vi "获得信号的最大幅值及对应的相位和频率.vi"(0 "信号":waveform(dbl)) -> (1 "max（f)":dbl, 2 "max幅值":dbl, 3 "max相位":dbl, 4 "幅值+ i相位":cdb)   [LabVIEW 2014]
uses:
  <vilib>/express/express analysis/Spectral/Block/exnSpectralBlock spectral measurements peak poly.vi
  <vilib>/express/express analysis/Spectral/Block/exnSpectralBlock spectral measurements peak WFM.vi
  <vilib>/express/express analysis/Spectral/XNode/ExpressSpectralMeasurementsBlockNode.xnode
panel:
  out "r":dbl
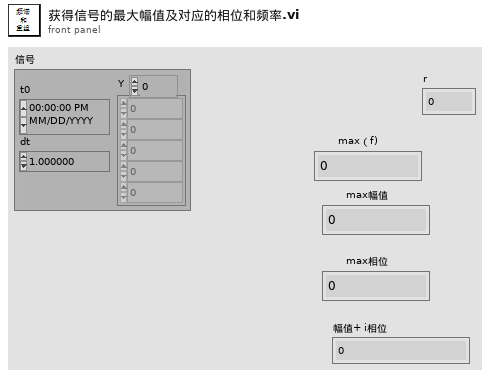
[diagram p1: front panel]
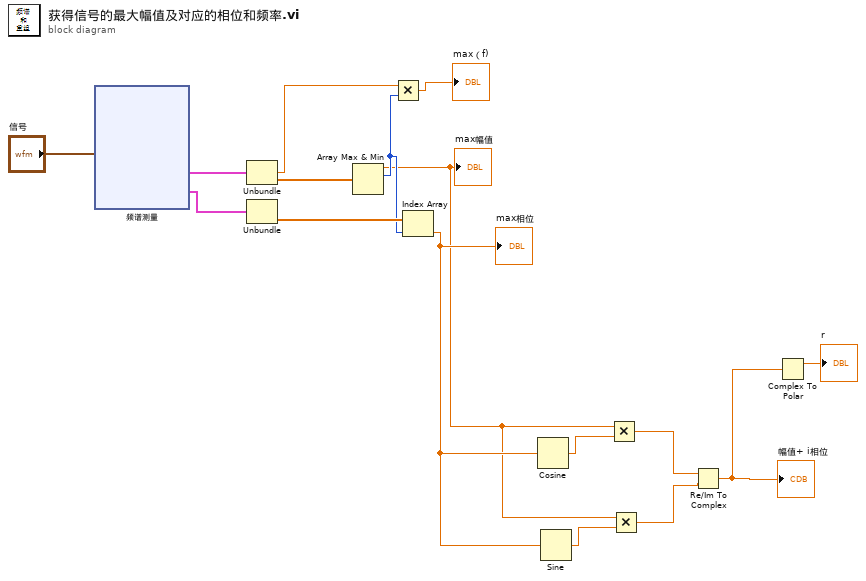
[diagram p0: block diagram]
diagram:
  n1 = xnode "频谱测量"("信号"="信号") -> ("FFT - （峰值）"=w16:cluster{"f0":dbl, "df":dbl, "magnitude":dbl[]}, "相位"=w15:cluster{"f0":dbl, "df":dbl, "phase":dbl[]})  [unwired: 1 in, 1 out]
  n2 = Unbundle(w16) -> ("df"=w13:dbl, "magnitude"=w14:dbl[])  [unwired: 1 out]
  n3 = Unbundle(w15) -> ("phase"=w11:dbl[])  [unwired: 2 out]
  n4 = Array Max & Min(array=w14) -> (max value=w6:dbl, max index (indices)=w10:i32)  [unwired: 2 out]
  "max幅值" <- w6
  n5 = Multiply(x=w13, y=w10) -> (x*y=→"max（f)":dbl)
  n6 = Index Array(array=w11, index=w10) -> (element=w9:dbl)
  "max相位" <- w9
  n7 = Cosine(x=w9) -> (cos(x)=w8:dbl)
  n8 = Sine(x=w9) -> (sin(x)=w7:dbl)
  n9 = Multiply(x=w6, y=w8) -> (x*y=w5:dbl)
  n10 = Multiply(x=w6, y=w7) -> (x*y=w4:dbl)
  n11 = Re/Im To Complex(1:w4, 2:w5) -> (0:w2:cdb)
  "幅值+ i相位" <- w2
  n12 = Complex To Polar(r * e^(i*theta)=w2) -> (r=→"r":dbl)  [unwired: 1 out]
